vi "Send Data.vi"(8 "error in (no error)":errorcluster, 10 "Data":T1={"M2 Dataset"={"Package"="", "Read Temp"=273.15, "Enable"=FALSE, "Piston"=FALSE, "Case Temp"=273.15, "Evap Temp"=273.15, "Feedback"=1, "TSD"=273.15, "Set Temp"=273.15}, "M1 Dataset"={"Package"="", "Read Temp"=273.15, "Enable"=FALSE, "Piston"=FALSE, "Case Temp"=273.15, "Evap Temp"=273.15, "Feedback"=1, "TSD"=273.15, "Set Temp"=273.15}, "Comp"=FALSE} {"M1 Dataset"."Set Temp" format="%.1f"; "M1 Dataset"."TSD" format="%.1f"; "M1 Dataset"."Feedback" items=["Evap Temp", "Case Temp", "Intec Temp", "TSD  Temp", "Autotune", "Extra"]; "M1 Dataset"."Evap Temp" format="%.1f"; "M1 Dataset"."Case Temp" format="%.1f"; "M1 Dataset"."Read Temp" format="%.1f"; "M2 Dataset"."Set Temp" format="%.1f"; "M2 Dataset"."TSD" format="%.1f"; "M2 Dataset"."Feedback" items=["Evap Temp", "Case Temp", "Intec Temp", "TSD  Temp", "Autotune", "Extra"]; "M2 Dataset"."Evap Temp" format="%.1f"; "M2 Dataset"."Case Temp" format="%.1f"; "M2 Dataset"."Read Temp" format="%.1f"}, 11 "Cobra RT in":refnum<class "Cobra RT.lvclass">) -> (0 "error out":errorcluster, 3 "Cobra RT out":refnum<class "Cobra RT.lvclass">)   [LabVIEW 2019]
uses:
  Test/Test Messages/NEA_Get Data Msg/NEA_Get Data Msg.lvclass
  Cobra RT.lvclass
  C:/Program Files (x86)/National Instruments/LabVIEW 2019/vi.lib/MGI/Panel Manager/Panel Actor/Panel Actor/Panel Actor.lvclass
  C:/Program Files (x86)/National Instruments/LabVIEW 2019/vi.lib/MGI/Monitored Actor/Monitored Actor/Monitored Actor/Monitored Actor.lvclass
  C:/Program Files (x86)/National Instruments/LabVIEW 2019/vi.lib/ActorFramework/Actor/Actor.lvclass
  <vilib>/ActorFramework/Message Enqueuer/Message Enqueuer.lvclass
panel:
  # "degC"
  # "degC"
  # "degC"
  # "degC"
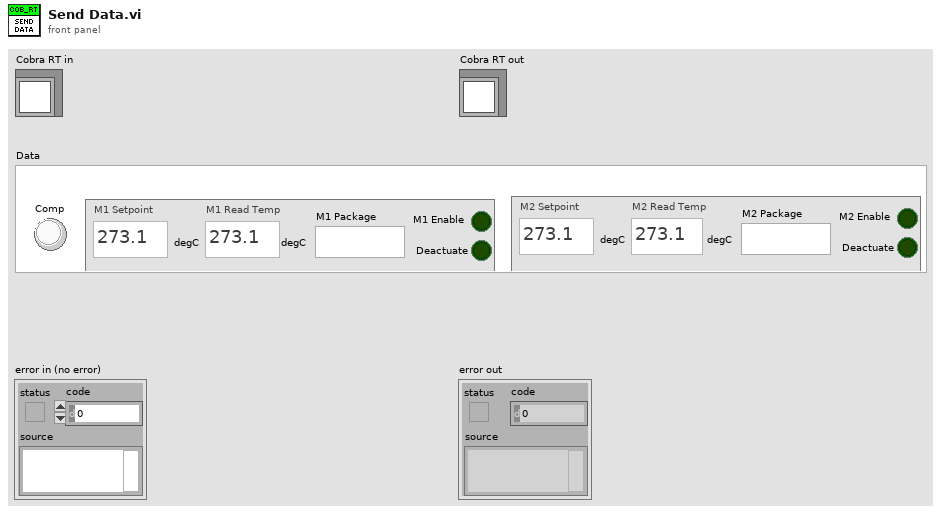
[diagram p1: front panel]
types:
  T1 = cluster{"M2 Dataset":cluster{"Package":string, "Read Temp":dbl, "Enable":bool, "Piston":bool, "Case Temp":dbl, "Evap Temp":dbl, "Feedback":u8, "TSD":dbl, "Set Temp":dbl}, "M1 Dataset":cluster{"Package":string, "Read Temp":dbl, "Enable":bool, "Piston":bool, "Case Temp":dbl, "Evap Temp":dbl, "Feedback":u8, "TSD":dbl, "Set Temp":dbl}, "Comp":bool}
  T2 = cluster{"M1 Dataset":cluster{"Package":string, "Set Temp":dbl[unit], "Read Temp":dbl[unit], "Enable":bool, "Piston":bool, "Case Temp":dbl[unit], "Evap Temp":dbl[unit], "Feedback":u8, "TSD":dbl[unit]}, "M2 Dataset":cluster{"Package":string, "Set Temp":dbl[unit], "Read Temp":dbl[unit], "Enable":bool, "Piston":bool, "Case Temp":dbl[unit], "Evap Temp":dbl[unit], "Feedback":u8, "TSD":dbl[unit]}, "Power":bool}
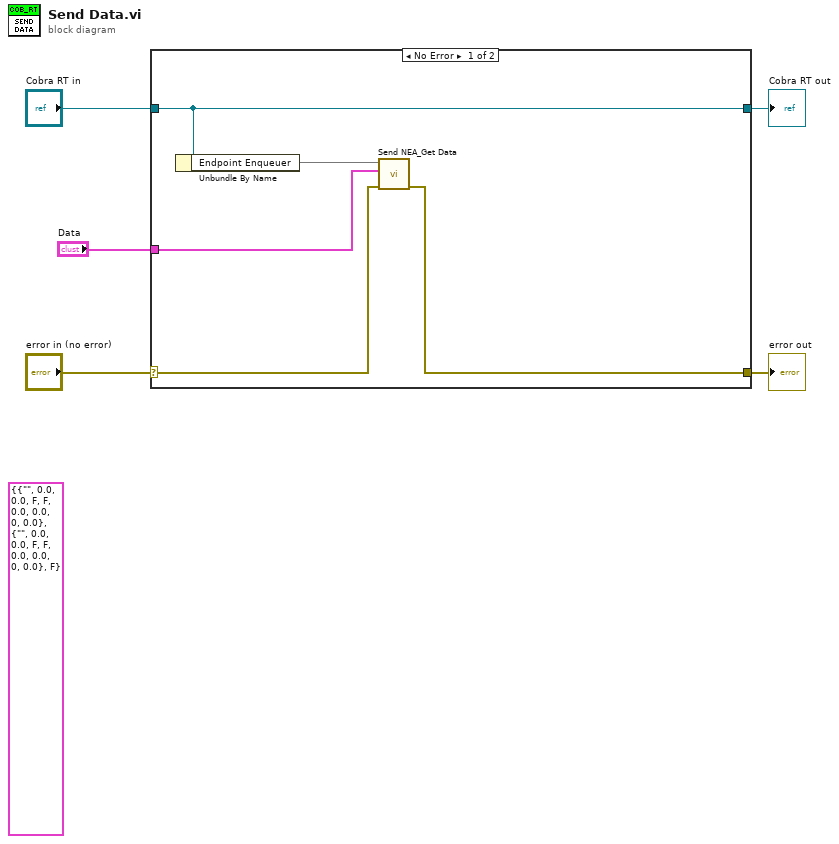
[diagram p0: block diagram]
diagram:
  (unwired) T2 {"M1 Dataset"={"Package"="", "Set Temp"=0.0, "Read Temp"=0.0, "Enable"=FALSE, "Piston"=FALSE, "Case Temp"=0.0, "Evap Temp"=0.0, "Feedback"=0, "TSD"=0.0}, "M2 Dataset"={"Package"="", "Set Temp"=0.0, "Read Temp"=0.0, "Enable"=FALSE, "Piston"=FALSE, "Case Temp"=0.0, "Evap Temp"=0.0, "Feedback"=0, "TSD"=0.0}, "Power"=FALSE} ("Data")
  n1 = case shown="No Error" "error in (no error)" {
    selector: "error in (no error)" -> [w7 w12]
    tunnel: [w6 w12] -> w4
    tunnel: [w10 w11] -> w2
    tunnel: "Cobra RT in" -> [w10 w11]
    tunnel: "Data" -> [w8 _]
    frame No Error {
      n2 = Unbundle By Name(w10) -> ("Endpoint Enqueuer"=w9)
      n3 = call "Send NEA_Get Data.vi"("error in (no error)"=w7, "Data"=w8, "Message Enqueuer"=w9) -> ("error out"=w6:errorcluster)  [unwired: 7 in, 1 out]
    }
    frame Error {
    }
  }
  "error out" <- w4
  "Cobra RT out" <- w2
